vi "PicoScope3000aSetupStreaming.vi"(0 "error in":errorcluster, 1 "Device Info":T2, 2 "handle in":i16, 3 "Acquisition Settings":T3={"Auto Stop"=FALSE, "Desired Sample Interval"=4, "Pre-trigger Samples"=0, "Post-trigger Samples"=1000, "Down-Sample Ratio"=1, "Down-Sample Mode"=0, "Time Units"=2} {"Time Units" items=["Nanoseconds (ns)"=2, "Microseconds (us)"=3, "Milliseconds (ms)"=4, "Seconds (s)"=5]; "Down-Sample Mode" items=["None"=0, "Aggregate"=1, "Decimate"=2, "Average"=4]}, 4 "Buffer and Transfer Settings":T1={"startIndex"=0, "Samples"=1000000, "Down Sample Ratio"=1, "Down-Sample Mode"=0} {"Down-Sample Mode" items=["None"=0, "Aggregate"=1, "Decimate"=2, "Average"=4]; "Down Sample Ratio" step=1; "Samples" format="%_6p"}, 5 "enabled array":i16[](array[numeric]), 6 "deviceIndex":u16, 10 "Pointers In":u64[][](array[numeric])) -> (11 "Pointer array":u64[][](array[numeric]), 14 "error out":errorcluster, 16 "handle out":i16, 17 "Sample Interval":u32, 19 "sampleIntervalTimeUnits":u32)   [LabVIEW 2010]
doc: "Set up the data buffers and calls RunStreaming to start the device streaming.\nData will be copied from the driver buffers into the corresponding application buffers using the wrapper dll."
uses:
  ps3000aWrap.dll
  ps3000a.dll
panel:
  # "Overview Buffer Size is the size of the temporary buffers used to\nstore data before returning it to the application."
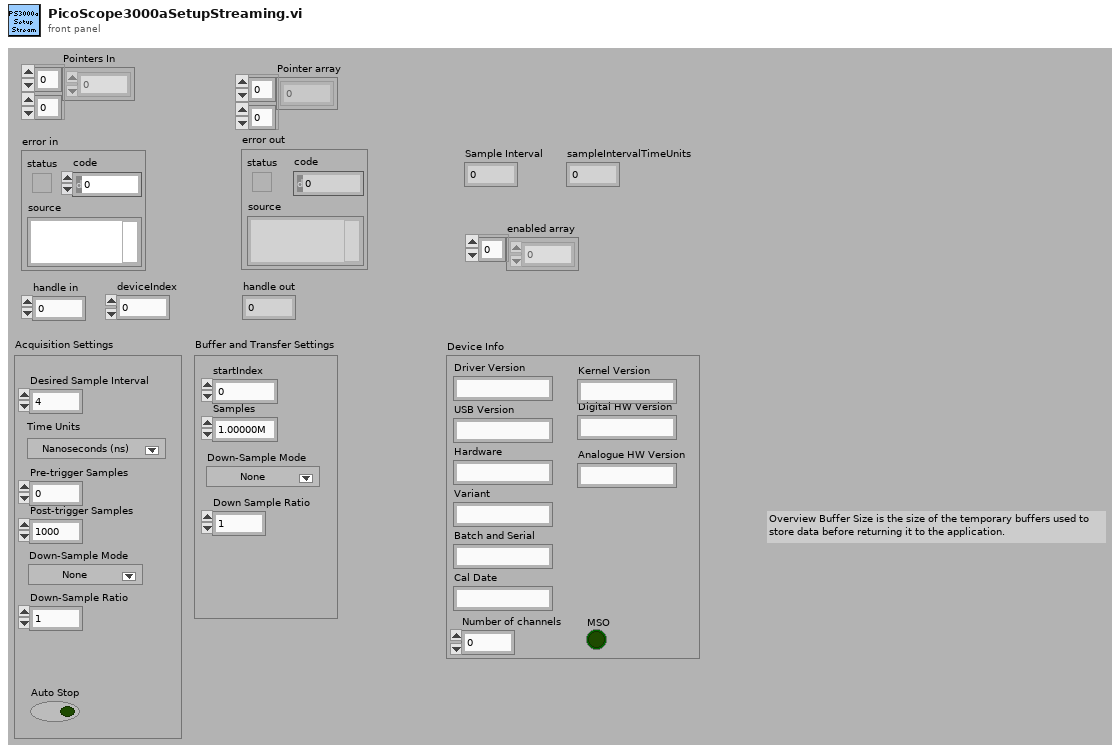
[diagram p1: front panel]
types:
  T1 = cluster{"startIndex":u64, "Samples":u64, "Down Sample Ratio":u64, "Down-Sample Mode":u32}
  T2 = cluster{"Driver Version":string, "USB Version":string, "Hardware":string, "Variant":string, "Batch and Serial":string, "Cal Date":string, "Kernel Version":string, "Digital HW Version":string, "Analogue HW Version":string, "MSO":bool, "Number of channels":i16}
  T3 = cluster{"Auto Stop":bool, "Desired Sample Interval":u32, "Pre-trigger Samples":u32, "Post-trigger Samples":u32, "Down-Sample Ratio":u32, "Down-Sample Mode":i32, "Time Units":u32}
  T4 = cluster{"status":bool, "code":u32, "source":string}
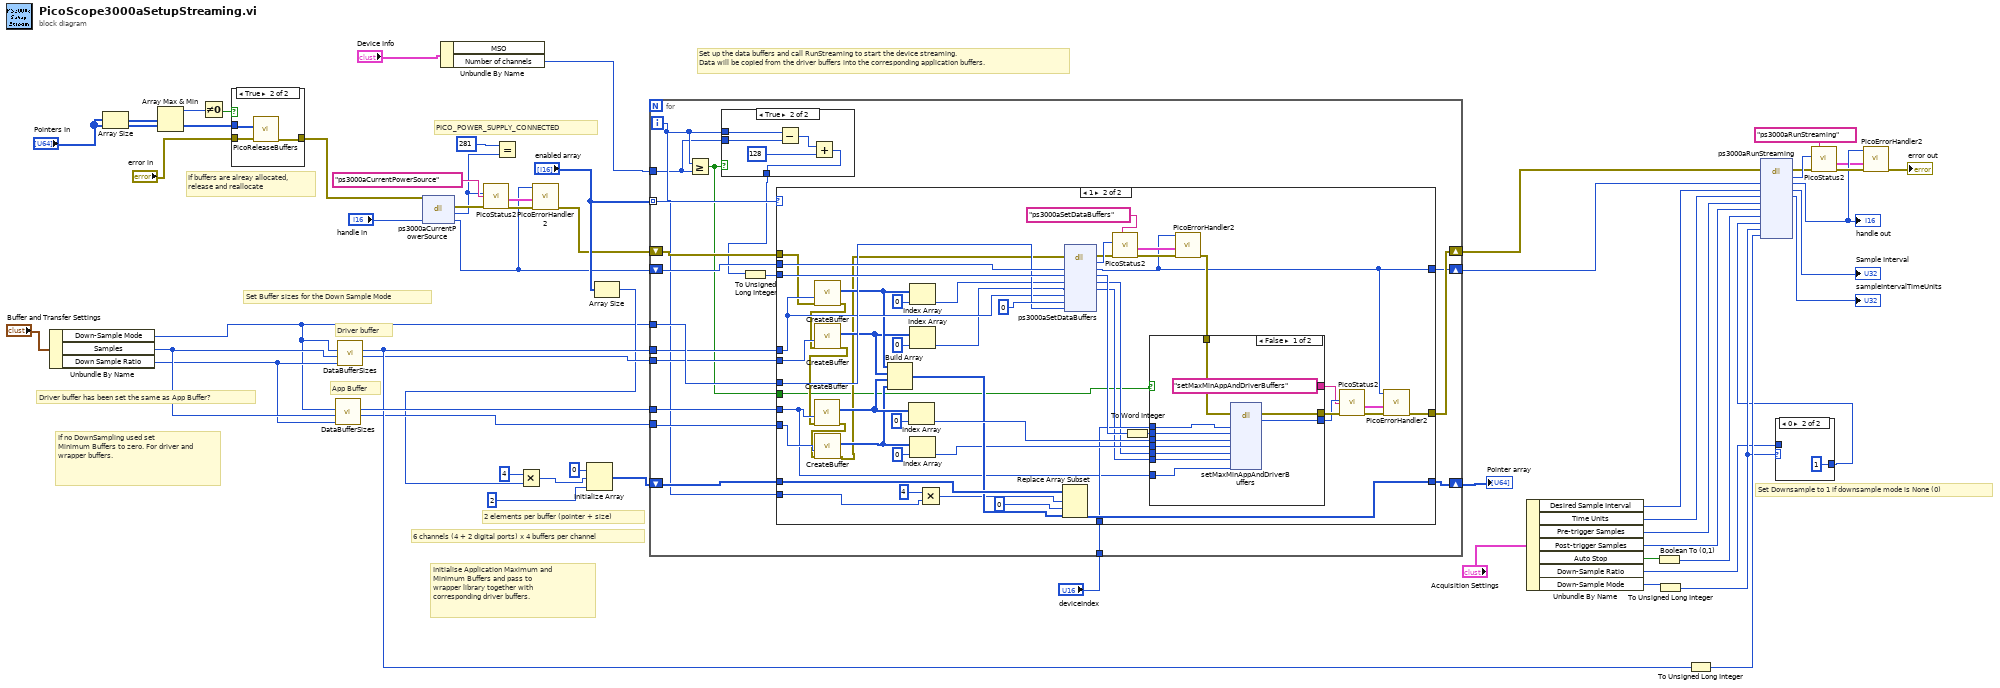
[diagram p0: block diagram]
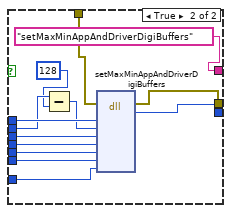
[diagram p6: hidden frame]
diagram:
  # "Set Downsample to 1 if downsample mode is None (0)"
  # "If buffers are alreay allocated,\nrelease and reallocate"
  # "2 elements per buffer (pointer + size)"
  # "6 channels (4 + 2 digital ports) x 4 buffers per channel"
  # "App Buffer"
  # "Driver buffer"
  # "Driver buffer has been set the same as App Buffer?"
  # "Set Buffer sizes for the Down Sample Mode"
  # "If no DownSampling used set \nMinimum Buffers to zero. For driver and wrapper buffers."
  # "PICO_POWER_SUPPLY_CONNECTED"
  # "Initialise Application Maximum and\nMinimum Buffers and pass to \nwrapper library together with corresponding driver buffers."
  # "Set up the data buffers and call RunStreaming to start the device streaming.\nData will be copied from the driver buffers into the corresponding application buffers."
  n1 = Unbundle By Name("Buffer and Transfer Settings") -> ("Down-Sample Mode"=w12:u32, "Samples"=w36:u64, "Down Sample Ratio"=w35:u64)
  n2 = Array Size(array="Pointers In") -> (size(s)=w15:i32[])
  n3 = Array Max & Min(array=w15) -> (max value=w14:i32)  [unwired: 3 out]
  n4 = Not Equal To 0?(x=w14) -> (x != 0?=w21:bool)
  n5 = case shown="True" w21 {
    tunnel: "Pointers In" -> [_ w59]
    tunnel: "error in" -> [w58 w60]
    tunnel: [w58 w61] -> w18
    frame False {
    }
    frame True {
      n6 = call "PicoReleaseBuffers.vi"("error in (no error)"=w60, "Pointer array"=w59) -> ("error out"=w61:errorcluster)  [unwired: 8 in, 1 out]
    }
  }
  n7 = call "DataBufferSizes.vi"("Down Sample Ratio"=w35, "Number of Samples"=w36, "Down-Sample Mode"=w12) -> ("min Buffer Size"=w31:i32, "Max Buffer Size"=w34:i32)  [unwired: 7 in]
  n8 = call "DataBufferSizes.vi"("Down Sample Ratio"=w35, "Number of Samples"=w36, "Down-Sample Mode"=w12) -> ("min Buffer Size"=w32:i32, "Max Buffer Size"=w33:i32)  [unwired: 7 in]
  n9 = dll-call lib="ps3000a.dll" fn="ps3000aCurrentPowerSource"(error in=w18, "handle"="handle in") -> (error out=w42:errorcluster, "PICO_STATUS"=w40:u32, "handle"=w2:i16)  [unwired: 2 in, 1 out]
  n10 = Unbundle By Name("Device Info") -> ("Number of channels"=w6:i16)  [unwired: 1 out]
  n11 = call "PicoStatus2.vi"("PICO source"="ps3000aCurrentPowerSource" ("source"), "Error in"=w42, "PICO STATUS"=w40) -> ("error out"=w5:errorcluster, "PICO_STATUS out"=w4:T4)  [unwired: 5 in]
  n12 = Equal?(x=u32 281, y=w40) -> ()  [unwired: 1 out]
  n13 = call "PicoErrorHandler2.vi"("error in (no error)"=w5, "PICO_STATUS in"=w4, "handle In"=w2) -> ("error out"=w3:errorcluster)  [unwired: 8 in]
  n14 = Array Size(array="enabled array") -> (size(s)=w25:i32)
  n15 = Multiply(x=4, y=w25) -> (x*y=w26:i32)
  n16 = Initialize Array(u64 0 ("element"), w26, 2 ("dimension size")) -> (w16:u64[][])
  n17 = for {
    tunnel: "enabled array" -> [w72] mode=indexing
    tunnel: w12 -> [w78]
    tunnel: w34 -> [w77]
    tunnel: w33 -> [w76]
    tunnel: w32 -> [w75]
    tunnel: w31 -> [w74]
    shift-right: [w71] -> w22
    shift-left: w3 -> [w70]
    shift-right: [w73] -> w30
    shift-left: w16 -> [w69]
    tunnel: "deviceIndex" -> [w66]
    shift-right: [w65] -> w7
    shift-left: w2 -> [w79]
    tunnel: w6 -> [w62]
    i -> [w64]
    n18 = Greater Or Equal?(x=w64, y=w62) -> (x >= y?=w63:bool)
    n19 = case shown="True" w63 {
      tunnel: [w80 w84] -> w67
      tunnel: w64 -> [w80 w82]
      tunnel: w62 -> [_ w81]
      frame False {
      }
      frame True {
        n20 = Subtract(x=w82, y=w81) -> (x-y=w83:i32)
        n21 = Add(x=w83, y=128) -> (x+y=w84:i32)
      }
    }
    n22 = To Unsigned Long Integer(number=w67) -> (unsigned 32bit integer=w68:u32)
    n23 = case shown="1" w72 {
      tunnel: w79 -> [w87 w139]
      tunnel: w70 -> [w86 w101]
      tunnel: w68 -> [_ w133]
      tunnel: w77 -> [_ w104]
      tunnel: w76 -> [_ w123]
      tunnel: w75 -> [_ w126]
      tunnel: w74 -> [_ w125]
      tunnel: w78 -> [_ w124]
      tunnel: w69 -> [w88 w117]
      tunnel: [w88 w116] -> w73
      tunnel: w64 -> [_ w113]
      tunnel: [w87 w89] -> w65
      tunnel: [w86 w90] -> w71
      tunnel: w66 -> [_ w105]
      tunnel: w63 -> [_ w96]
      frame 0, Default {
      }
      frame 1 {
        n24 = call "CreateBuffer.vi"("error in (no error)"=w101, "Buffer size"=w123) -> ("error out"=w100:errorcluster, "Pointer and BufferSize"=w121:u64[])  [unwired: 8 in]
        n25 = call "CreateBuffer.vi"("error in (no error)"=w100, "Buffer size"=w126) -> ("error out"=w99:errorcluster, "Pointer and BufferSize"=w120:u64[])  [unwired: 8 in]
        n26 = call "CreateBuffer.vi"("error in (no error)"=w99, "Buffer size"=w104) -> ("error out"=w98:errorcluster, "Pointer and BufferSize"=w119:u64[])  [unwired: 8 in]
        n27 = call "CreateBuffer.vi"("error in (no error)"=w98, "Buffer size"=w125) -> ("error out"=w97:errorcluster, "Pointer and BufferSize"=w118:u64[])  [unwired: 8 in]
        n28 = Build Array(w121, w120, w119, w118) -> (w112:u64[][])
        n29 = Index Array(array=w119, index=0) -> (element=w122:u64)
        n30 = Index Array(array=w121, index=0) -> (element=w115:u64)
        n31 = Index Array(array=w120, index=0) -> (element=w106:u64)
        n32 = Index Array(array=w118, index=0) -> (element=w107:u64)
        n33 = Multiply(x=4, y=w113) -> (x*y=w111:i32)
        n34 = Replace Array Subset(array=w117, new element=w112, index (row)=w111, index (col)=0 ("disabled index (row)")) -> (w116:u64[][])
        n35 = dll-call lib="ps3000a.dll" fn="ps3000aSetDataBuffers" ("ps3000.dll:_ps3000_open_unit@0")(error in=w97, "handle"=w139, "channel"=w133, "bufferMax"=w115, "bufferMin"=w106, "bufferLth"=w123, "segmentIndex"=u32 0, "downSampleRatioMode"=w124) -> (error out=w137:errorcluster, "PICO_STATUS"=w138:u32, "handle"=w89:i16, "channel"=w134:u32, "bufferMax"=w103:u64, "bufferMin"=w102:u64)  [unwired: 5 in, 1 out]
        n36 = call "PicoStatus2.vi"("PICO source"="ps3000aSetDataBuffers" ("source"), "Error in"=w137, "PICO STATUS"=w138) -> ("error out"=w109:errorcluster, "PICO_STATUS out"=w93:T4)  [unwired: 5 in]
        n37 = To Word Integer(number=w134) -> (16bit integer=w135:i16)
        n38 = call "PicoErrorHandler2.vi"("error in (no error)"=w109, "PICO_STATUS in"=w93, "handle In"=w89) -> ("error out"=w108:errorcluster)  [unwired: 8 in]
        n39 = case shown="False" w96 {
          tunnel: w135 -> [w150 w153]
          tunnel: [w149 w158] -> w132
          tunnel: [w148 w157] -> w131
          tunnel: w122 -> [w147 w162]
          tunnel: w103 -> [w146 w160]
          tunnel: w108 -> [w145 w163]
          tunnel: w107 -> [w144 w161]
          tunnel: w102 -> [w143 w159]
          tunnel: w105 -> [w142 w155]
          tunnel: w104 -> [w141 w156]
          tunnel: ["setMaxMinAppAndDriverBuffers" ("source") "setMaxMinAppAndDriverDigiBuffers" ("source")] -> w95
          frame False {
            n40 = dll-call lib="ps3000aWrap.dll" fn="setMaxMinAppAndDriverBuffers"(error in=w145, "deviceIndex"=w142, "channel"=w150, "appMaxBuffer"=w147, "appMinBuffer"=w144, "driverMaxBuffer"=w146, "driverMinBuffer"=w143, "bufferLength"=w141) -> (error out=w149:errorcluster, "status"=w148:u32)  [unwired: 9 in, 1 out]
          }
          frame True {
            n41 = Subtract(x=w153, y=i16 128) -> (x-y=w154:i16)
            n42 = dll-call lib="ps3000aWrap.dll" fn="setMaxMinAppAndDriverDigiBuffers"(error in=w163, "deviceIndex"=w155, "digiport"=w154, "appMaxDigiBuffer"=w162, "appMinDigiBuffer"=w161, "driverMaxDigiBuffer"=w160, "driverMinDigiBuffer"=w159, "bufferLength"=w156) -> (error out=w158:errorcluster, "PICO STATUS"=w157:u32)  [unwired: 9 in, 1 out]
          }
        }
        n43 = call "PicoStatus2.vi"("PICO source"=w95, "Error in"=w132, "PICO STATUS"=w131) -> ("error out"=w92:errorcluster, "PICO_STATUS out"=w91:T4)  [unwired: 5 in]
        n44 = call "PicoErrorHandler2.vi"("error in (no error)"=w92, "PICO_STATUS in"=w91, "handle In"=w89) -> ("error out"=w90:errorcluster)  [unwired: 8 in]
      }
    }
  }
  "Pointer array" <- w30
  n45 = Unbundle By Name("Acquisition Settings") -> ("Desired Sample Interval"=w50:u32, "Time Units"=w44:u32, "Pre-trigger Samples"=w49:u32, "Post-trigger Samples"=w48:u32, "Auto Stop"=w47:bool, "Down-Sample Ratio"=w10:u32, "Down-Sample Mode"=w45:i32)
  n46 = Boolean To (0,1)(Boolean=w47) -> (0, 1=w51:i16)
  n47 = To Unsigned Long Integer(number=w45) -> (unsigned 32bit integer=w11:u32)
  n48 = To Unsigned Long Integer(number=w33) -> (unsigned 32bit integer=w13:u32)
  n49 = case shown="0" w11 {
    tunnel: [w164 u32 1 ("Down-Sample Ratio")] -> w9
    tunnel: w10 -> [w164 _]
    frame Default {
    }
    frame 0 {
    }
  }
  n50 = dll-call lib="ps3000a.dll" fn="ps3000aRunStreaming" ("ps5000a.dll:_ps3000_open_unit@0")(error in=w22, "handle"=w7, "sampleInterval"=w50, "sampleIntervalTimeUnits"=w44, "maxPreTriggerSamples"=w49, "maxPostTriggerSamples"=w48, "autoStop"=w51, "downSampleRatio"=w9, "downSampleRatioMode"=w11, "overviewBufferSize"=w13) -> (error out=w55:errorcluster, "PICO_STATUS"=w56:u32, "handle"=w17:i16, "sampleInterval"=→"Sample Interval":u32, "sampleIntervalTimeUnits"=→"sampleIntervalTimeUnits":u32)  [unwired: 8 in, 1 out]
  "handle out" <- w17
  n51 = call "PicoStatus2.vi"("PICO source"="ps3000aRunStreaming" ("source"), "Error in"=w55, "PICO STATUS"=w56) -> ("error out"=w53:errorcluster, "PICO_STATUS out"=w1:T4)  [unwired: 5 in]
  n52 = call "PicoErrorHandler2.vi"("error in (no error)"=w53, "PICO_STATUS in"=w1, "handle In"=w17) -> ("error out"=→"error out":errorcluster)  [unwired: 8 in]
